vi "REG - Display2DTrain.vi"(8 "error in":errorcluster, 11 "Local":T5={"Parameters"={"Plot"=refnum, "Data"={"Split"={"X Train"=[], "X Test"=[], "Y Train"=[], "Y Test"=[]}, "Predict"=[]}, "Display"={"Choice"=enum."All", "Indexe"={"X"=0, "Y"=1}}, "Point Property"={"Train Style"=enum."Full circle", "Test OK Style"=enum."Full square", "Label Color"=[8978528, 4367871, 16716800], "Test NO OK"={"Style"=enum."Cross", "Color"=16711680}}, "Tolerance's threshold"=0.0}, "2D Array"=[], "Point ID"=[], "GoodPredict"=0, "Rating 2D Array"=[]}) -> (0 "error out":errorcluster, 3 "Local_Out":T5={"Parameters"={"Plot"=refnum, "Data"={"Split"={"X Train"=[], "X Test"=[], "Y Train"=[], "Y Test"=[]}, "Predict"=[]}, "Display"={"Choice"=enum."All", "Indexe"={"X"=0, "Y"=1}}, "Point Property"={"Train Style"=enum."Full circle", "Test OK Style"=enum."Full square", "Label Color"=[8978528, 4367871, 16716800], "Test NO OK"={"Style"=enum."Cross", "Color"=16711680}}, "Tolerance's threshold"=0.0}, "2D Array"=[], "Point ID"=[], "GoodPredict"=0, "Rating 2D Array"=[]})   [LabVIEW 2020]
uses:
  _Controls/Datas.ctl
  _Controls/PointPropertyMultipleLabel.ctl
  _Controls/Style.ctl
  _Controls/2DData.ctl
types:
  T1 = typedef "Datas.ctl" = cluster{"Split":cluster{"X Train":dbl[][], "X Test":dbl[][], "Y Train":dbl[][], "Y Test":dbl[][]}, "Predict":dbl[][]}
  T2 = typedef "PointPropertyMultipleLabel.ctl" = cluster{"Train Style":T3, "Test OK Style":T3, "Label Color":u32[], "Test NO OK":cluster{"Style":T3, "Color":u32}}
  T3 = typedef "Style.ctl" = enum16{"Empty circle", "Full circle", "Empty square", "Full square", "Cross"}
  T4 = typedef "2DData.ctl" = cluster{"Tag":i32, "X":dbl[], "Y":dbl[]}
  T5 = cluster{"Parameters":cluster{"Plot":refnum<vi>, "Data":T1, "Display":cluster{"Choice":enum16{"All", "Train", "Test"}, "Indexe":cluster{"X":i32, "Y":i32}}, "Point Property":T2, "Tolerance's threshold":dbl}, "2D Array":cluster{"X":dbl[], "Y":dbl[]}[], "Point ID":cluster{"DataUse":enum16{"Dataset", "Train", "Test"}, "Color":u32}[], "GoodPredict":i32, "Rating 2D Array":T4[]}
  T6 = cluster{"DataUse":enum16{"Dataset", "Train", "Test"}, "Color":u32}[]
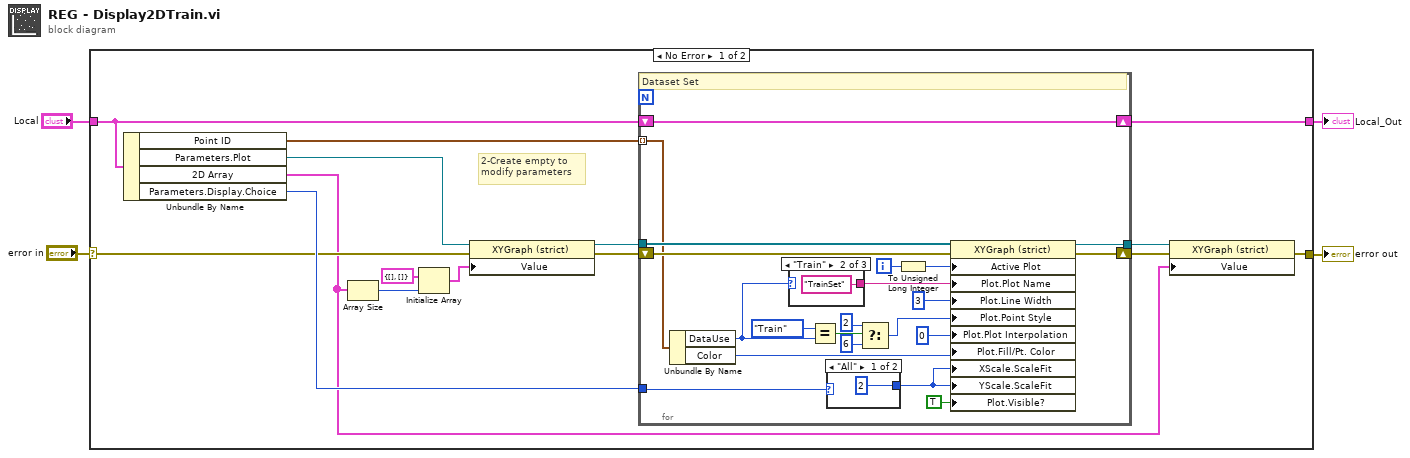
[diagram p0: block diagram]
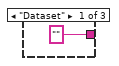
[diagram p2: hidden frame]
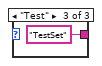
[diagram p3: hidden frame]
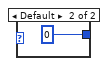
[diagram p4: hidden frame]
diagram:
  n1 = case shown="No Error" "error in" {
    selector: "error in" -> [w8 w47]
    tunnel: "Local" -> [w17 w46]
    tunnel: [w10 w47] -> w4
    tunnel: [w14 w46] -> w1
    frame No Error {
      # "2-Create empty to \nmodify parameters"
      n2 = Unbundle By Name(w17) -> ("Point ID"=w7:T6, "Parameters.Plot"=w5:refnum<vi>, "2D Array"=w6:cluster{"X":dbl[], "Y":dbl[]}[], "Parameters.Display.Choice"=w9:enum16{"All", "Train", "Test"})
      n3 = Array Size(array=w6) -> (size(s)=w13:i32)
      n4 = Initialize Array(cluster{dbl[], dbl[]} {[], []}, w13) -> (w18:cluster{dbl[], dbl[]}[])
      n5 = property class="XYGraph (strict)"(reference=w5, error in=w8, "Value"=w18) -> (reference out=w15:refnum<vi>, error out=w16:errorcluster)
      n6 = for {
        tunnel: w15 -> [w40]
        tunnel: w7 -> [w33] mode=indexing
        shift-right: [w28] -> w14
        shift-left: w17 -> [w28]
        tunnel: [w26] -> w12
        shift-right: [w36] -> w11
        shift-left: w16 -> [w39]
        tunnel: w9 -> [w25]
        i -> [w35]
        # "Dataset Set"
        n7 = Unbundle By Name(w33) -> ("DataUse"=w21:enum16{"Dataset", "Train", "Test"}, "Color"=w27:u32)
        n8 = case shown="\"Train\"" w21 {
          tunnel: ["" "TrainSet" "TestSet"] -> w22
          frame "Dataset" {
          }
          frame "Train" {
          }
          frame "Test" {
          }
        }
        n9 = Equal?(x=enum16{"Dataset", "Train", "Test"}."Train", y=w21) -> (x = y?=w32:bool)
        n10 = case shown="\"All\"" w25 {
          tunnel: [u8 2 ("X Scale.Scale Fit") u8 0 ("X Scale.Scale Fit")] -> w24
          frame "All" {
          }
          frame Default {
          }
        }
        n11 = Select(t=u8 2 ("Plot.Point Style"), s=w32, f=u8 6 ("Plot.Point Style")) -> (s? t:f=w29:u8)
        n12 = To Unsigned Long Integer(number=w35) -> (unsigned 32bit integer=w34:u32)
        n13 = property class="XYGraph (strict)"(reference=w40, error in=w39, "Active Plot"=w34, "Plot.Plot Name"=w22, "Plot.Line Width"=u8 3, "Plot.Point Style"=w29, "Plot.Plot Interpolation"=u8 0, "Plot.Fill/Pt. Color"=w27, "XScale.ScaleFit"=w24, "YScale.ScaleFit"=w24, "Plot.Visible?"=TRUE ("Plot.Visible")) -> (reference out=w26:refnum<vi>, error out=w36:errorcluster)
      }
      n14 = property class="XYGraph (strict)"(reference=w12, error in=w11, "Value"=w6) -> (error out=w10:errorcluster)  [unwired: 1 out]
    }
    frame Error {
    }
  }
  "error out" <- w4
  "Local_Out" <- w1
